vi "KE622x -- Setup DC Current Source Example.vi"() -> ()   [LabVIEW 2019, in "Keithley 622x.lvlib"]
doc: "Example VI showing how to source a DC current."
uses:
  Keithley 622x.lvlib
  Configure/Source/Typedefs/KE622x -- Current Range.ctl
  Configure/Source/Typedefs/KE622x -- Current Ranges.ctl
  Typedefs/KE622x -- On Off Control.ctl
  Utility/Typedefs/KE622x -- Instrument Type.ctl
  Configure/Output/Typedefs/KE6221 -- Output Response.ctl
  Configure/Source/Typedefs/KE622x -- Current Level.ctl
  Configure/Source/Typedefs/KE622x -- Voltage Limit.ctl
panel:
  in  "Output State":T1
  out "error out":errorcluster
  in  "Turn Off Output If Voltage Limit?":bool=TRUE
  out "Voltage Limit?":bool
  out "Interlock Tripped?":bool
  in  "Voltage Limit (V)":T2=10.0 min=0.1 max=105.0 step=0.01 format="%.2p"
  in  "Current Level (A)":T3=0.001 min=-0.105 max=0.105 format="%.4p"
  in  "Output Response":T4=enum."Slow"
  in  "Instrument Type":T5=enum."KE6221"
  in  "Analog Filter State":T1
  in  "Current Range In":T6={"Auto Range?"=TRUE, "Man / Selected\nRange"=enum."2nA"}
  in  "Check For SCPI Errors? (T)":bool=TRUE
  in  "VISA resource name":refnum<visa-resource-name>
  # "Input"
  # "Output"
  # "*** NOTE:  only apples to KE6221"
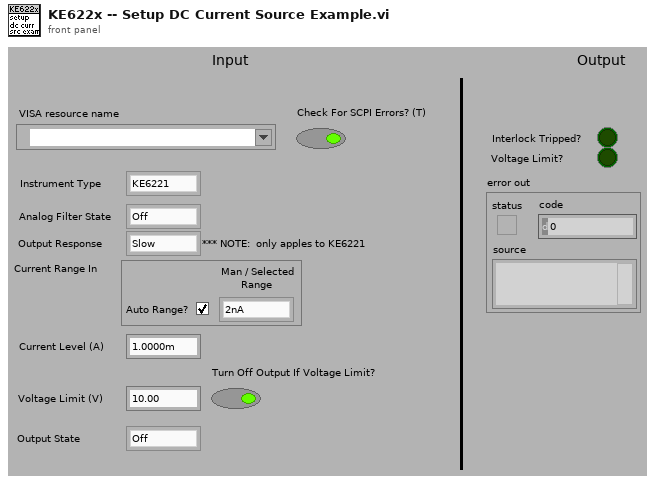
[diagram p1: front panel]
types:
  T1 = typedef "Keithley 622x.lvlib/KE622x -- On Off Control.ctl" = enum16{"Off", "On"}
  T2 = typedef "Keithley 622x.lvlib/KE622x -- Voltage Limit.ctl" = dbl
  T3 = typedef "Keithley 622x.lvlib/KE622x -- Current Level.ctl" = dbl
  T4 = typedef "Keithley 622x.lvlib/KE6221 -- Output Response.ctl" = enum16{"Fast", "Slow"}
  T5 = typedef "Keithley 622x.lvlib/KE622x -- Instrument Type.ctl" = enum16{"KE6220", "KE6221"}
  T6 = typedef "Keithley 622x.lvlib/KE622x -- Current Range.ctl" = cluster{"Auto Range?":bool, "Man / Selected\nRange":T7}
  T7 = typedef "Keithley 622x.lvlib/KE622x -- Current Ranges.ctl" = enum16{"2nA", "20nA", "200nA", "2uA", "20uA", "200uA", "2mA", "20mA", "100mA"}
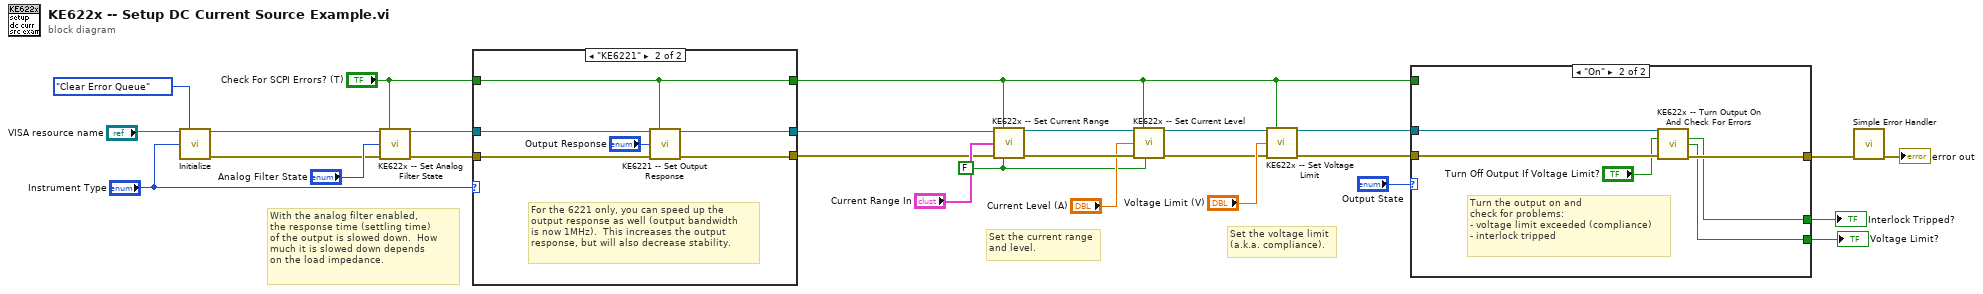
[diagram p0: block diagram]
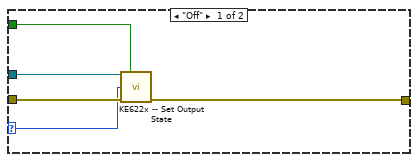
[diagram p2: hidden frame]
diagram:
  w12 = FALSE ("Read Back Set Values? (T)")
  # "Set the voltage limit\n(a.k.a. compliance)."
  # "Set the current range\nand level."
  # "With the analog filter enabled,\nthe response time (settling time)\nof the output is slowed down.  How\nmuch it is slowed down depends\non the load impedance."
  n1 = call "Initialize.vi"("VISA resource name"="VISA resource name", "Error Queue Option"=enum16{"Clear Error Queue", "Error Query"}."Clear Error Queue", "Instrument Type"="Instrument Type") -> ("VISA resource name out"=w23:refnum<visa-resource-name>, "error out"=w22:errorcluster)  [unwired: 11 in]
  n2 = call "KE622x -- Set Analog Filter State.vi"("Resource In"=w23, "Check For SCPI Errors? (T)"="Check For SCPI Errors? (T)", "Analog Filter State"="Analog Filter State", "error in (no error)"=w22) -> ("Resource Out (dupl)"=w21:refnum<visa-resource-name>, "error out"=w19:errorcluster)  [unwired: 10 in]
  n3 = case shown="\"KE6221\"" "Instrument Type" {
    tunnel: w21 -> [w29 w36]
    tunnel: w19 -> [w28 w34]
    tunnel: [w29 w33] -> w16
    tunnel: "Check For SCPI Errors? (T)" -> [w30 w32]
    tunnel: [w30 w32] -> w3
    tunnel: [w28 w31] -> w17
    frame "KE6220" {
    }
    frame "KE6221" {
      # "For the 6221 only, you can speed up the\noutput response as well (output bandwidth\nis now 1MHz).  This increases the output\nresponse, but will also decrease stability."
      n4 = call "KE6221 -- Set Output Response.vi"("Resource In"=w36, "Check For SCPI Errors? (T)"=w32, "KE6221 Output Response"="Output Response", "error in (no error)"=w34) -> ("Resource Out (dupl)"=w33:refnum<visa-resource-name>, "error out"=w31:errorcluster)  [unwired: 10 in]
    }
  }
  n5 = call "KE622x -- Set Current Range.vi"("Resource In"=w16, "Check For SCPI Errors? (T)"=w3, "Current Range In"="Current Range In", "error in (no error)"=w17, "Read Back Set Values? (T)"=w12) -> ("Resource Out (dupl)"=w15:refnum<visa-resource-name>, "error out"=w14:errorcluster)  [unwired: 8 in, 1 out]
  n6 = call "KE622x -- Set Current Level.vi"("Resource In"=w15, "Check For SCPI Errors? (T)"=w3, "Current Level (A) In"="Current Level (A)", "error in (no error)"=w14, "Read Back Set Value? (T)"=w12) -> ("Resource Out (dupl)"=w10:refnum<visa-resource-name>, "error out"=w9:errorcluster)  [unwired: 8 in, 1 out]
  n7 = call "KE622x -- Set Voltage Limit.vi"("Resource In"=w10, "Check For SCPI Errors? (T)"=w3, "Voltage Limit (V)"="Voltage Limit (V)", "error in (no error)"=w9) -> ("Resource Out (dupl)"=w8:refnum<visa-resource-name>, "error out"=w7:errorcluster)  [unwired: 10 in]
  n8 = case shown="\"On\"" "Output State" {
    selector: "Output State" -> [w39 _]
    tunnel: w8 -> [w41 w47]
    tunnel: w7 -> [w40 w46]
    tunnel: [w37 w44] -> w6
    tunnel: w3 -> [w38 _]
    tunnel: [_ w43] -> w2
    tunnel: [_ w42] -> w1
    frame "Off" {
      n9 = call "KE622x -- Set Output State.vi"("Resource In"=w41, "Check For SCPI Errors? (T)"=w38, "Output State"=w39, "error in (no error)"=w40) -> ("error out"=w37:errorcluster)  [unwired: 10 in, 1 out]
    }
    frame "On" {
      # "Turn the output on and\ncheck for problems:\n- voltage limit exceeded (compliance)\n- interlock tripped"
      n10 = call "KE622x -- Turn Output On And Check For Errors.vi"("Resource In"=w47, "Turn Off Output If Compliance?"="Turn Off Output If Voltage Limit?", "error in (no error)"=w46) -> ("Interlock Tripped?"=w43:bool, "Compliance?"=w42:bool, "error out"=w44:errorcluster)  [unwired: 9 in, 1 out]
    }
  }
  "Interlock Tripped?" <- w2
  "Voltage Limit?" <- w1
  n11 = call <vilib>:"Simple Error Handler.vi"("error in (no error)"=w6) -> ("error out"=→"error out":errorcluster)  [unwired: 4 in, 4 out]
